vi "Wingbeat Amplitude Extraction (Host).vi"(0 "NumWingSectors":u8, 1 "Wing ROIs":T1) -> ()   [LabVIEW 2013, in "Image Processing.lvlib"]
uses:
  Image Processing.lvlib
  <vilib>/rvi/interface/nirviReadWriteControl/nirviReadWriteControl.xnode
  <vilib>/rvi/interface/Simulation/niFpgaSimulationCallBeginRW.vi
  <vilib>/rvi/errors/niLvFpgaAdjustHostInterfaceError.vi
  <vilib>/rvi/interface/nirviMethod/nirviMethod.xnode
  <vilib>/rvi/interface/nirviOpenFPGA/nirviOpenFPGA.xnode
  FPGA Bitfiles/10-Tap8-bitwith_DRAM.lvbitx
  <vilib>/FPGAPlugInAG/Dynamic/niLvFpga_Reset_Dynamic.vi
  <vilib>/FPGAPlugInAG/Dynamic/niLvFpga_Run_Dynamic.vi
  <vilib>/rvi/interface/nirviCloseFPGA/nirviCloseFPGA.xnode
  <vilib>/FPGAPlugInAG/Dynamic/niLvFpga_Close_Dynamic.vi
  <vilib>/FPGAPlugInAG/PCIe-1473R/niLvFpga_Open_PCIe-1473R.vi
  <vilib>/rvi/interface/common/dynamic/niFpgaDynamicAddResources.vi
  <vilib>/userdefined/High Color/nirio_resource_hc.ctl
panel:
  in  "Signal Mapping":T2(ring)=enum."Basler 10-tap"
  in  "Line Scan":bool
  in  "RIO Device":T3="RIO0"
  in  "Start Serial Server":bool=TRUE
  out "Acq'd Frame Height":u32=1088
  out "Frames Acq'd":u32=1
  out "Acq'd Frame Width":u32=2040
  in  "Stopped":bool=TRUE
  out "Acq In Progress":bool
  in  "Acquire":bool
  in  "Frames To Acquire":u32=1 caption="Frames To Acquire\n(0 = infinite)"
  in  "Stop":bool
  in  "Cancel":bool
  out "Initialized":bool
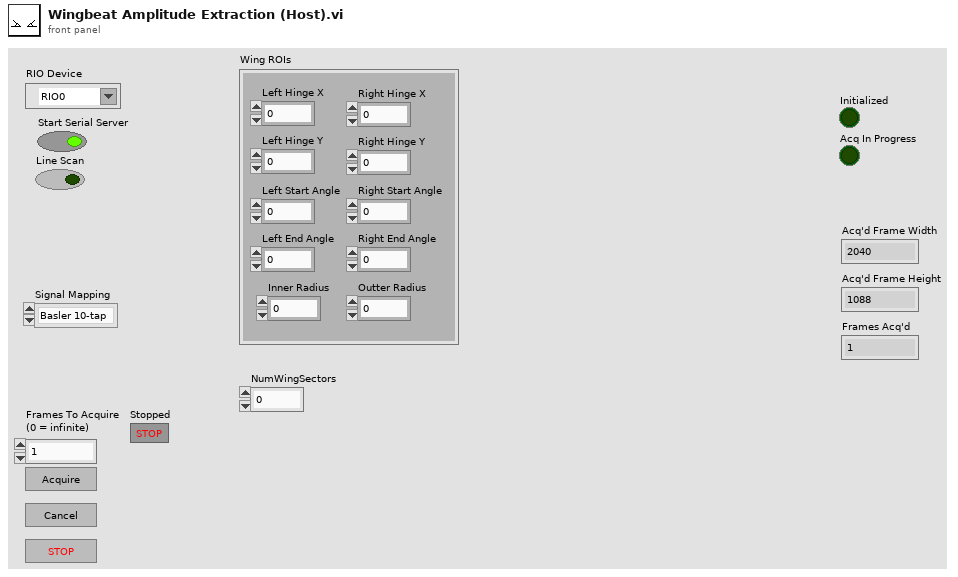
[diagram p1: front panel]
types:
  T1 = cluster{"Left Hinge X":u16, "Left Hinge Y":u16, "Inner Radius":u16, "Outter Radius":u16, "Right Hinge X":u16, "Right Hinge Y":u16, "Right Start Angle":i16, "Right End Angle":i16, "Left Start Angle":i16, "Left End Angle":i16}
  T2 = enum8{"Standard", "Basler 10-tap", "Vosskühler 10-tap"}
  T3 = typedef "nirio_resource_hc.ctl" = tag
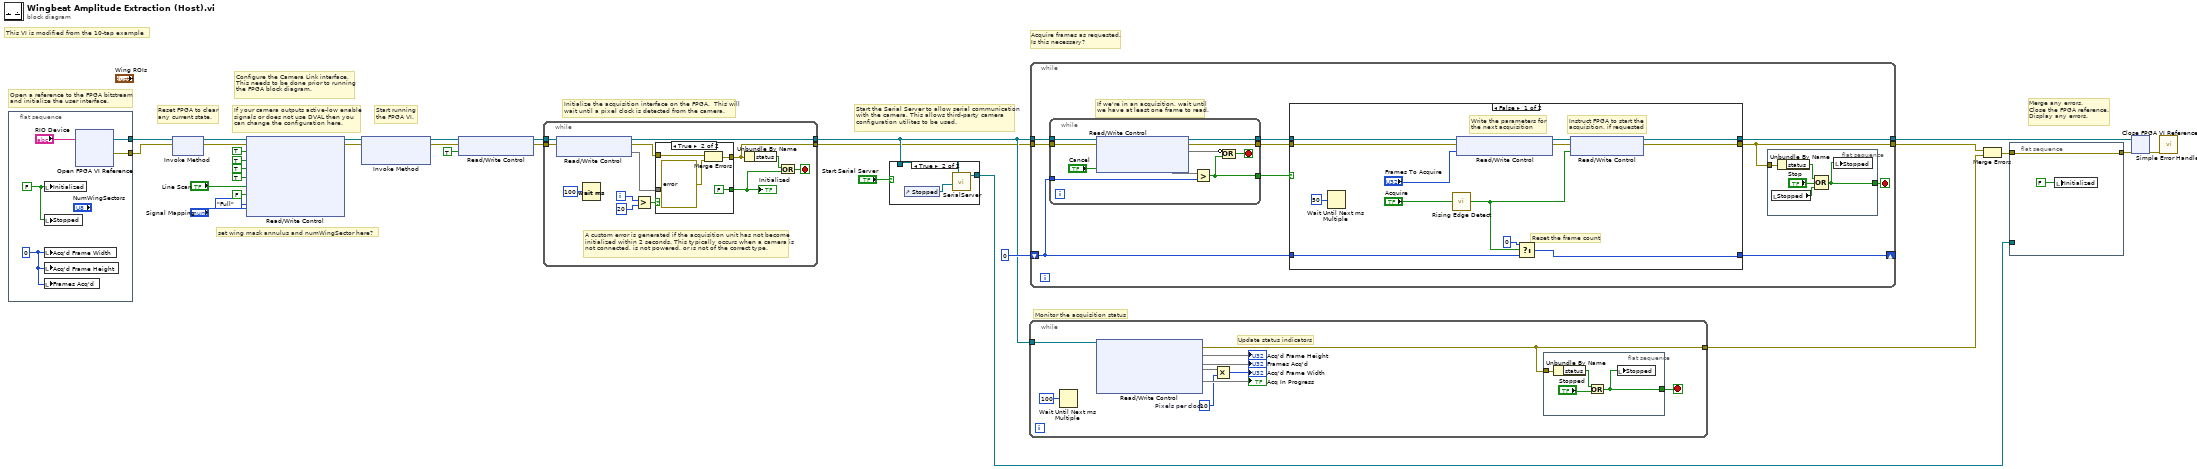
[diagram p0: block diagram]
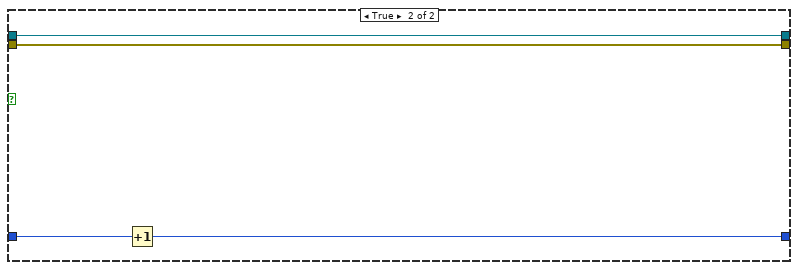
[diagram p3: hidden frame]
diagram:
  # "This VI is modified from the 10-tap example"
  # "set wing mask annulus and numWingSector here?"
  # "If your camera outputs active-low enable\nsignals or does not use DVAL then you \ncan change the configuration here."
  # "Start running\nthe FPGA VI."
  # "Reset FPGA to clear\nany current state."
  # "Merge any errors.\nClose the FPGA reference.\nDisplay any errors."
  # "Acquire frames as requested.\nIs this necessary?"
  # "Monitor the acquisition status"
  # "Start the Serial Server to allow serial communication\nwith the camera. This allows third-party camera\nconfiguration utilites to be used."
  # "Initialize the acquisition interface on the FPGA.  This will\nwait until a pixel clock is detected from the camera."
  # "Configure the Camera Link interface.\nThis needs to be done prior to running\nthe FPGA block diagram."
  # "Open a reference to the FPGA bitstream\nand initialize the user interface."
  n1 = flat-sequence {
    tunnel: [w33] -> w22
    tunnel: [w32] -> w30
    frame #0 {
      w35 = u32 0 ("Num Lines Acq'd")
      w31 = FALSE ("stop")
      n2 = local write "Initialized"(w31) -> ()
      n3 = local write "Stopped"(w31) -> ()
      n4 = local write "Acq'd Frame Width"(w35) -> ()
      n5 = local write "Acq'd Frame Height"(w35) -> ()
      n6 = local write "Frames Acq'd"(w35) -> ()
      n7 = xnode "Open FPGA VI Reference"("resource name"="RIO Device") -> ("FPGA VI Reference Out"=w33:refnum<k20>, "error out"=w32:errorcluster)  [unwired: 1 in]
    }
  }
  n8 = xnode "Invoke Method"("FPGA VI Reference In"=w22, "error in"=w30) -> ("FPGA VI Reference Out"=w14:refnum<k20>, "error out"=w17:errorcluster)
  n9 = xnode "Read/Write Control"("FPGA VI Reference In"=w14, "error in"=w17, "CL Config.FVAL Active High"=TRUE ("IO Module Config.CL FVAL Active High"), "CL Config.LVAL Active High"=TRUE ("IO Module Config.CL LVAL Active High"), "CL Config.DVAL Active High"=TRUE ("IO Module Config.CL DVAL Active High"), "CL Config.Spare Active High"=TRUE ("IO Module Config.CL Spare Active High"), "CL Config.Line Scan"="Line Scan", "Acq Control.Ignore DVAL"=FALSE ("CL Config.Line Scan"), "CL Config.Configuration"=enum8{"Base", "Medium", "Full"}."Full", "CL Config.Signal Mapping"="Signal Mapping") -> ("FPGA VI Reference Out"=w18:refnum<k20>, "error out"=w16:errorcluster)
  n10 = xnode "Invoke Method"("FPGA VI Reference In"=w18, "error in"=w16) -> ("FPGA VI Reference Out"=w3:refnum<k20>, "error out"=w2:errorcluster)  [unwired: 1 in]
  n11 = xnode "Read/Write Control"("FPGA VI Reference In"=w3, "error in"=w2, "Acq Control.Initialize"=TRUE ("Arm Acquisition")) -> ("FPGA VI Reference Out"=w29:refnum<k20>, "error out"=w28:errorcluster)
  n12 = while {
    tunnel: w29 -> [w43]
    tunnel: w28 -> [w42]
    tunnel: [w41] -> w8
    tunnel: [w45] -> w1
    i -> [w37]
    stop <- w48 stop-if-true
    # "A custom error is generated if the acquisition unit has not become\ninitialized within 2 seconds. This typically occurs when a camera is\nnot connected, is not powered, or is not of the correct type."
    n13 = xnode "Read/Write Control"("FPGA VI Reference In"=w43, "error in"=w42) -> ("FPGA VI Reference Out"=w41:refnum<k20>, "error out"=w40:errorcluster, "Acq Status.Initialized"=w39)
    n14 = Wait (ms)(milliseconds to wait=u32 100) -> ()  [unwired: 1 out]
    n15 = Greater?(x=w37, y=20) -> (0:w38:bool)
    n16 = case shown="True" w38 {
      tunnel: [w50 FALSE] -> w44
      tunnel: w39 -> [w50 _]
      tunnel: w40 -> [w49 w52]
      tunnel: [w49 w54] -> w45
      frame False {
      }
      frame True {
        n17 = Merge Errors(w52, errorcluster {"status"=TRUE, "code"=-8999, "source"="Acquisition Initialization: This error typically occurs when a camera is not properly connected, is not powered, or is not of the correct type."} ("error in")) -> (w54:errorcluster)
      }
    }
    "Initialized" <- w44
    n18 = Unbundle By Name(w45) -> ("status"=w47:bool)
    n19 = Or(x=w47, y=w44) -> (x .or. y?=w48:bool)
  }
  n20 = case shown="True" "Start Serial Server" {
    tunnel: [_ w55] -> w23
    tunnel: w8 -> [_ w56]
    frame False {
    }
    frame True {
      n21 = control-ref of="Stopped"() -> (w57:refnum<vi>)
      n22 = call "SerialServer.vi"("Stop Refnum"=w57, 7:w56) -> ("FPGA VI Reference Out"=w55:refnum<k20>)  [unwired: 4 in, 1 out]
    }
  }
  n23 = while {
    tunnel: w8 -> [w65]
    tunnel: [w58] -> w19
    stop <- w67 stop-if-true
    w59 = u32 10  # Pixels per clock
    # "Update status indicators"
    n24 = Wait Until Next ms Multiple(millisecond multiple=u32 100) -> ()  [unwired: 1 out]
    n25 = xnode "Read/Write Control"("FPGA VI Reference In"=w65) -> ("error out"=w58:errorcluster, "Acq Status.Lines Per Frame"=→"Acq'd Frame Height", "Acq Status.Frames Acq'd"=→"Frames Acq'd", "Acq Status.Clocks Per Line"=w60, "Acq Status.Acq In Progress"=→"Acq In Progress")  [unwired: 1 in, 2 out]
    n26 = Multiply(x=w60, y=w59) -> (x*y=→"Acq'd Frame Width":u32)
    n27 = flat-sequence {
      tunnel: w58 -> [w71]
      tunnel: [w69] -> w67
      frame #0 {
        n28 = Unbundle By Name(w71) -> ("status"=w70:bool)
        n29 = Or(x=w70, y="Stopped") -> (x .or. y?=w69:bool)
        n30 = local write "Stopped"(w69) -> ()
      }
    }
  }
  n31 = while {
    tunnel: w8 -> [w78]
    tunnel: w1 -> [w77]
    tunnel: [w80] -> w20
    tunnel: [w81] -> w27
    shift-right: [w73] -> _
    shift-left: u32 0 -> [w72]
    stop <- w79 stop-if-true
    # "If we're in an acquisition, wait until\nwe have at least one frame to read."
    n32 = while {
      tunnel: w78 -> [w88]
      tunnel: w77 -> [w87]
      tunnel: [w85] -> w76
      tunnel: [w86] -> w75
      tunnel: w72 -> [w91]
      tunnel: [w89] -> w74
      stop <- w90 stop-if-true
      n33 = xnode "Read/Write Control"("FPGA VI Reference In"=w88, "error in"=w87, "Acq Control.Cancel Acq"="Cancel") -> ("FPGA VI Reference Out"=w86:refnum<k20>, "error out"=w85:errorcluster, "Acq Status.Acq In Progress"=w84, "Acq Status.Frames Acq'd"=w83)
      n34 = Greater?(x=w83, y=w91) -> (0:w89:bool)
      n35 = Compound Arithmetic op=OR(invert w84, w89) -> (w90:bool)
    }
    n36 = case shown="False" w74 {
      tunnel: w75 -> [w106 w111]
      tunnel: w76 -> [w105 w110]
      tunnel: [w101 w110] -> w80
      tunnel: [w104 w111] -> w81
      tunnel: w72 -> [w107 w113]
      tunnel: [w109 w112] -> w73
      frame False {
        # "Reset the frame count"
        # "Instruct FPGA to start the\nacquisition, if requested"
        # "Write the parameters for\nthe next acquisition"
        n37 = Wait Until Next ms Multiple(millisecond multiple=u32 50) -> ()  [unwired: 1 out]
        n38 = call "Rising Edge Detect.vi"("Input"="Acquire") -> ("Pulse"=w97:bool)  [unwired: 4 in]
        n39 = xnode "Read/Write Control"("FPGA VI Reference In"=w106, "error in"=w105, "Acq Control.Frames To Acq"="Frames To Acquire") -> ("FPGA VI Reference Out"=w103:refnum<k20>, "error out"=w102:errorcluster)
        n40 = Select(t=u32 0, s=w97, f=w107) -> (s? t:f=w109:u32)
        n41 = xnode "Read/Write Control"("FPGA VI Reference In"=w103, "error in"=w102, "Acq Control.Acquire"=w97) -> ("FPGA VI Reference Out"=w104:refnum<k20>, "error out"=w101:errorcluster)
      }
      frame True {
        n42 = Increment(x=w113) -> (x+1=w112:u32)
      }
    }
    n43 = flat-sequence {
      tunnel: w80 -> [w94]
      tunnel: [w93] -> w79
      frame #0 {
        n44 = local read "Stopped"() -> (w92:bool)
        n45 = Unbundle By Name(w94) -> ("status"=w95:bool)
        n46 = Compound Arithmetic op=OR(w95, "Stop", w92) -> (w93:bool)
        n47 = local write "Stopped"(w93) -> ()
      }
    }
  }
  n48 = Merge Errors(w20, w19) -> (w21:errorcluster)
  n49 = flat-sequence {
    tunnel: w21 -> [w115]
    tunnel: [w115] -> w26
    tunnel: w23 -> [_]
    frame #0 {
      n50 = local write "Initialized"(FALSE ("Module Enabled")) -> ()
    }
  }
  n51 = xnode "Close FPGA VI Reference"("FPGA VI Reference In"=w27, "error in"=w26) -> ("error out"=w24:errorcluster)
  n52 = call <vilib>:"Simple Error Handler.vi"("error in (no error)"=w24) -> ()  [unwired: 4 in, 5 out]
